vi "windows_mouse_event.vi"(5 "Left up":bool, 7 "Left down":bool, 8 "error in (no error)":errorcluster, 10 "y":i32, 11 "x":i32) -> (0 "error out":errorcluster, 3 "vi path (only on error)":path)   [LabVIEW 2011]
uses:
  user32.dll
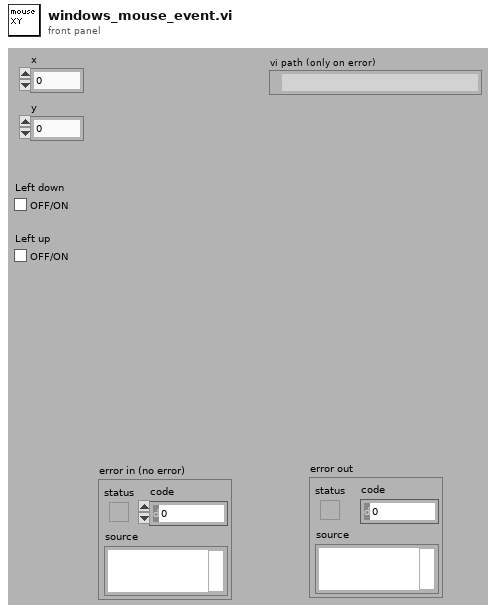
[diagram p1: front panel]
types:
  T1 = typedef "LVRectTypeDef.ctl" = cluster{"left":i16, "top":i16, "right":i16, "bottom":i16}
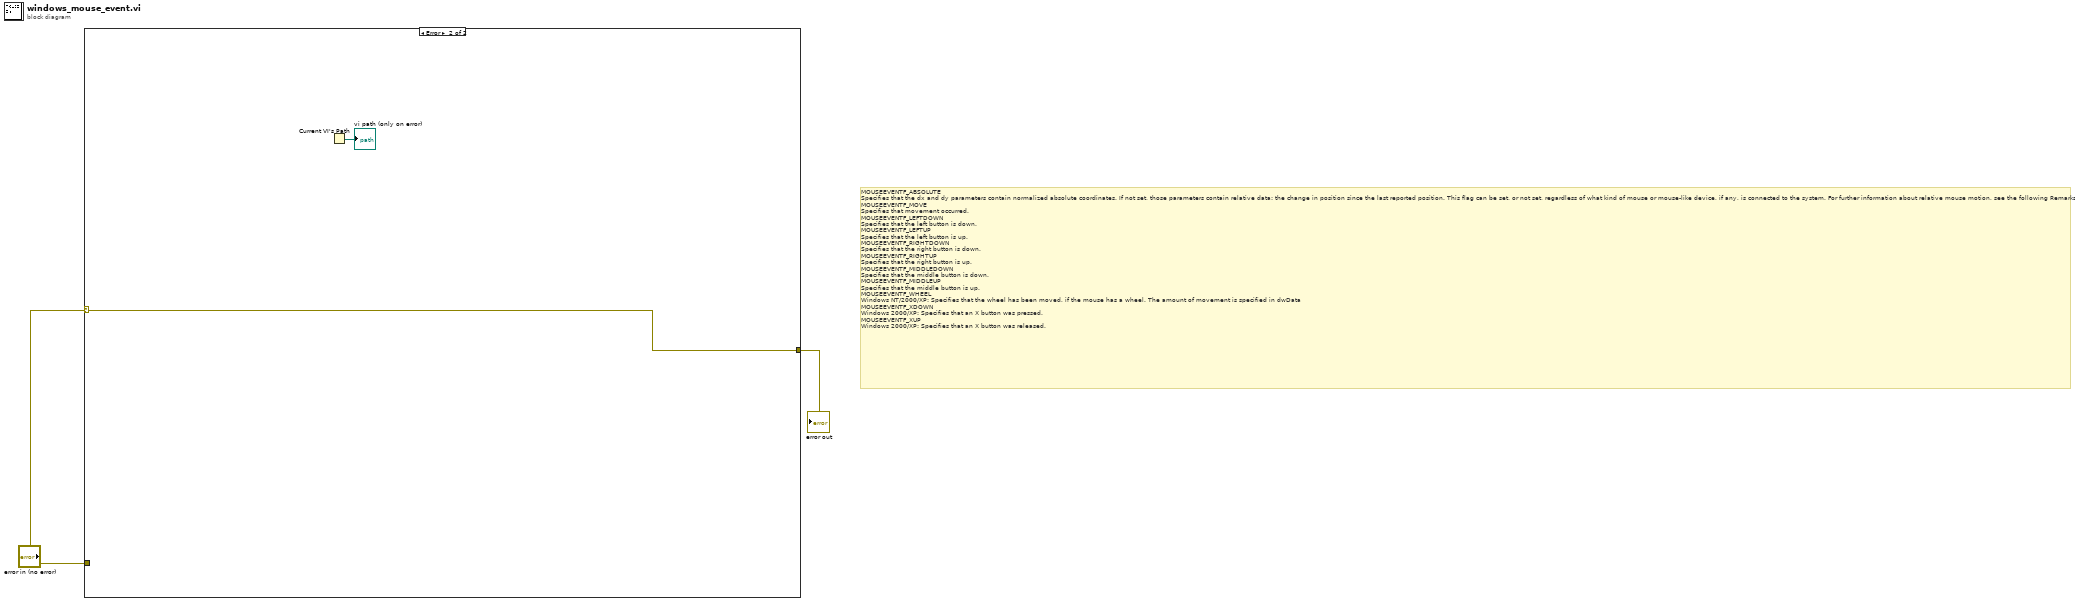
[diagram p0: block diagram]
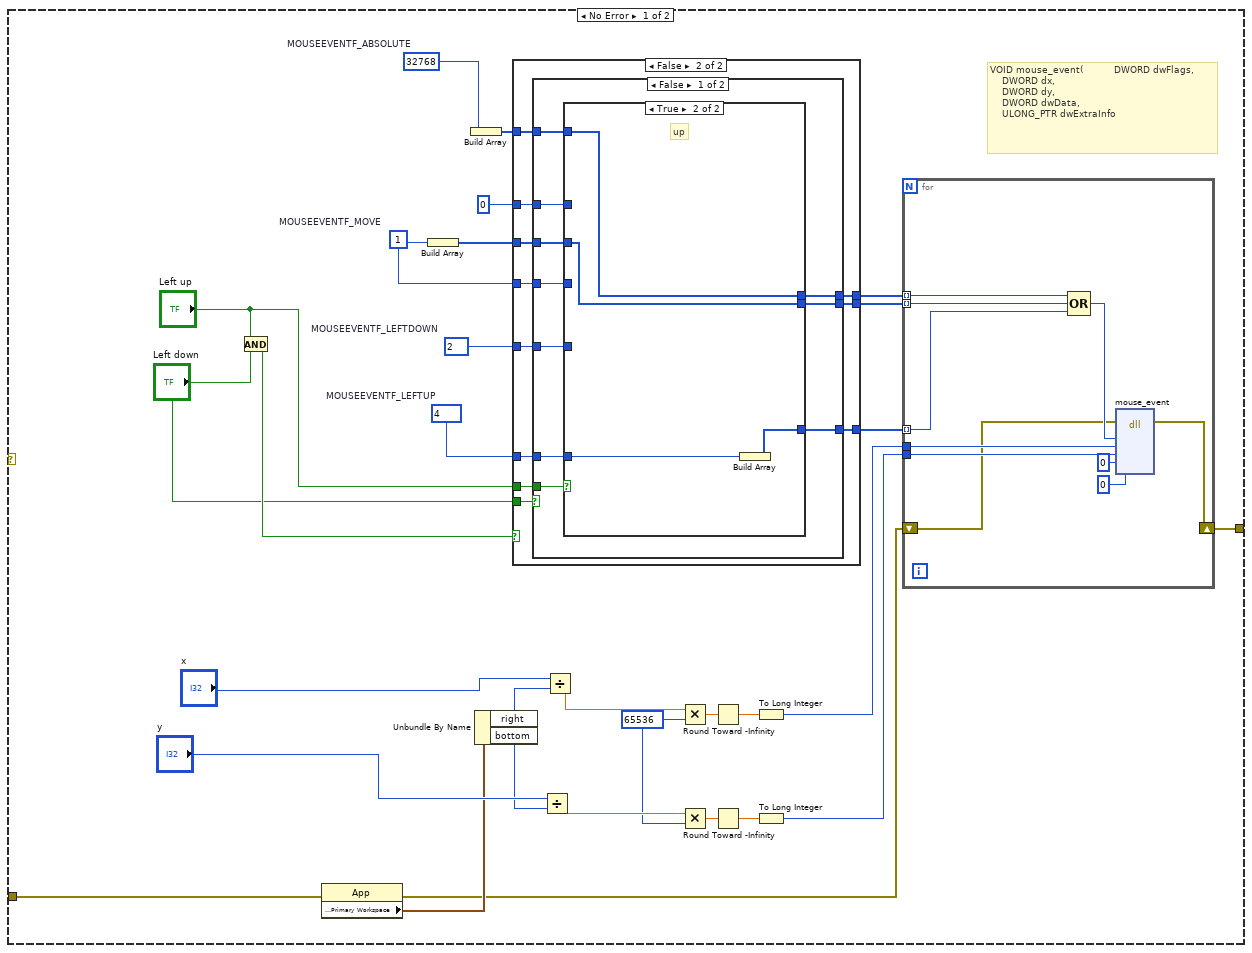
[diagram p2: hidden frame]
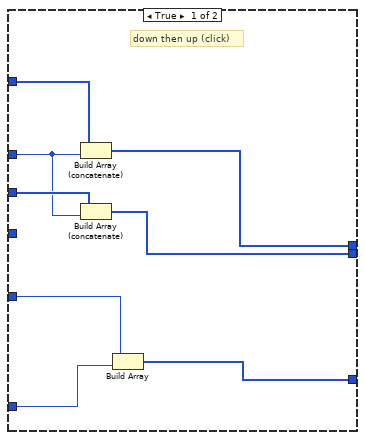
[diagram p3: hidden frame]
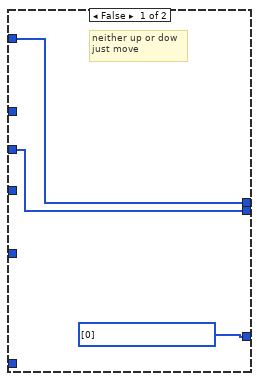
[diagram p4: hidden frame]
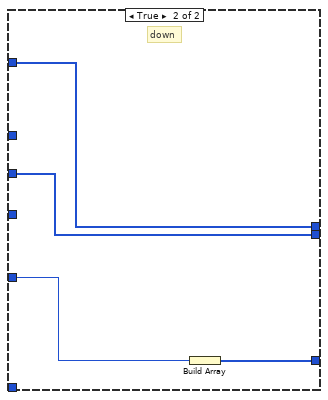
[diagram p5: hidden frame]
diagram:
  # "MOUSEEVENTF_ABSOLUTE\nSpecifies that the dx and dy parameters contain normalized absolute coordinates. If not set, those parameters contain relative data: the change in position since the last reported position. This flag can be set, or not set, regardless of what kind of mouse or mouse-like device, if any, is connected to the system. For further information about relative mouse motion, see the following Remarks section.\nMOUSEEVENTF_MOVE\nSpecifies that movement occurred.\nMOUSEEVENTF_LEFTDOWN\nSpecifies that the left button is down.\nMOUSEEVENTF_LEFTUP\nSpecifies that the left button is up.\nMOUSEEVENTF_RIGHTDOWN\nSpecifies that the right button is down.\nMOUSEEVENTF_RIGHTUP\nSpecifies that the right button is up.\nMOUSEEVENTF_MIDDLEDOWN\nSpecifies that the middle button is down.\nMOUSEEVENTF_MIDDLEUP\nSpecifies that the middle button is up.\nMOUSEEVENTF_WHEEL\nWindows NT/2000/XP: Specifies that the wheel has been moved, if the mouse has a wheel. The amount of movement is specified in dwData\nMOUSEEVENTF_XDOWN\nWindows 2000/XP: Specifies that an X button was pressed.\nMOUSEEVENTF_XUP\nWindows 2000/XP: Specifies that an X button was released."
  n1 = case shown="Error" "error in (no error)" {
    selector: "error in (no error)" -> [_ w84]
    tunnel: "error in (no error)" -> [w23 _]
    tunnel: [w12 w84] -> w2
    frame No Error {
      w21 = 2  # MOUSEEVENTF_LEFTDOWN
      w22 = 4  # MOUSEEVENTF_LEFTUP
      w4 = 65536 ("y")
      w26 = 1  # MOUSEEVENTF_MOVE
      w17 = 32768  # MOUSEEVENTF_ABSOLUTE
      # "VOID mouse_event(          DWORD dwFlags,\n    DWORD dx,\n    DWORD dy,\n    DWORD dwData,\n    ULONG_PTR dwExtraInfo"
      n2 = And(x="Left up", y="Left down") -> (x .and. y?=w16:bool)
      n3 = property class="App"(error in=w23) -> (error out=w13:errorcluster, "Display:Primary Workspace"=w20:T1)  [unwired: 1 in, 1 out]
      n4 = Build Array(w26) -> (w29:i32[])
      n5 = Build Array(w17) -> (w30:i32[])
      n6 = Unbundle By Name(w20) -> ("right"=w19:i16, "bottom"=w18:i16)
      n7 = case shown="False" w16 {
        tunnel: [w48 w53] -> w32
        tunnel: w22 -> [w49 w56]
        tunnel: w21 -> [w50 w57]
        tunnel: [w46 w55] -> w31
        tunnel: w30 -> [w47 w61]
        tunnel: 0 ("f") -> [w43 w60]
        tunnel: w29 -> [w45 w59]
        tunnel: [w44 w54] -> w27
        tunnel: w26 -> [_ w58]
        tunnel: "Left down" -> [_ w52]
        tunnel: "Left up" -> [_ w51]
        frame True {
          # "down then up (click)"
          n8 = Build Array (concatenate)(w47, w43) -> (w46:i32[])
          n9 = Build Array (concatenate)(w45, w43) -> (w44:i32[])
          n10 = Build Array(w50, w49) -> (w48:i32[])
        }
        frame False {
          n11 = case shown="False" w52 {
            tunnel: [w66 w82] -> w53
            tunnel: w56 -> [w63 _]
            tunnel: w57 -> [w67 w81]
            tunnel: [w64 w80] -> w55
            tunnel: w61 -> [w71 w80]
            tunnel: w60 -> [w70 _]
            tunnel: w59 -> [w69 w79]
            tunnel: [w65 w79] -> w54
            tunnel: w58 -> [w68 _]
            tunnel: w51 -> [w62 _]
            frame False {
              n12 = case shown="True" w62 {
                tunnel: [i32[] [0] w78] -> w66
                tunnel: w63 -> [_ w77]
                tunnel: w67 -> [_ _]
                tunnel: [w73 w76] -> w64
                tunnel: w71 -> [w73 w76]
                tunnel: w70 -> [_ _]
                tunnel: w69 -> [w72 w75]
                tunnel: [w72 w75] -> w65
                tunnel: w68 -> [_ _]
                frame False {
                  # "neither up or dow\njust move"
                }
                frame True {
                  # "up"
                  n13 = Build Array(w77) -> (w78:i32[])
                }
              }
            }
            frame True {
              # "down"
              n14 = Build Array(w81) -> (w82:i32[])
            }
          }
        }
      }
      n15 = Divide(x="y", y=w18) -> (x/y=w5:dbl)
      n16 = Divide(x="x", y=w19) -> (x/y=w10:dbl)
      n17 = Multiply(x=w10, y=w4) -> (x*y=w9:dbl)
      n18 = Multiply(x=w5, y=w4) -> (x*y=w7:dbl)
      n19 = Round Toward -Infinity(1:w9) -> (0:w11:dbl)
      n20 = Round Toward -Infinity(1:w7) -> (0:w6:dbl)
      n21 = To Long Integer(number=w11) -> (32bit integer=w8:i32)
      n22 = To Long Integer(number=w6) -> (32bit integer=w3:i32)
      n23 = for {
        tunnel: w31 -> [w39] mode=indexing
        tunnel: w32 -> [w38] mode=indexing
        tunnel: w27 -> [w37] mode=indexing
        tunnel: w3 -> [w36]
        tunnel: w8 -> [w35]
        shift-right: [w34] -> w12
        shift-left: w13 -> [w33]
        n24 = Compound Arithmetic op=OR(w39, w37, w38) -> (w40:i32)
        n25 = dll-call lib="user32.dll" fn="mouse_event"(error in=w33, "dwFlags"=w40, "dx"=w35, "dy"=w36, "dwData"=0, "dwExtraInfo"=0) -> (error out=w34:errorcluster)  [unwired: 7 in, 2 out]
      }
    }
    frame Error {
      n26 = Current VI's Path() -> (path=→"vi path (only on error)":path)
    }
  }
  "error out" <- w2
